vi "LIA Example RT.vi"() -> ()   [LabVIEW 2017]
uses:
  lib/rt/example/Lock-In Amplifier Example RT.lvclass
  <vilib>/userdefined/High Color/nirio_resource_hc.ctl
  lib/rt/example/Properties/Server_GET.vi
  lib/rt/example/Properties/FpgaSession_GET.vi
  lib/rt/server/RT FlexRIO Server TCP.lvclass
  lib/interface/Interface FPGA/LIA Host Interface FPGA.lvclass
panel:
  out "Initialized":bool
  in  "stop":bool
  out "error out":errorcluster
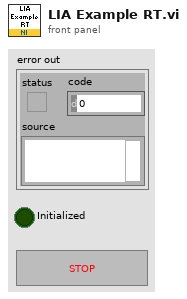
[diagram p1: front panel]
types:
  T1 = typedef "nirio_resource_hc.ctl" = tag
  T2 = typedef "Lock-In Amplifier Example Shared.lvlib/message.ctl" = cluster{"command":u32, "payload":string}
  T3 = typedef "RT FlexRIO Server TCP.lvclass/connection state.ctl" = enum16{"started", "connected", "stopped"}
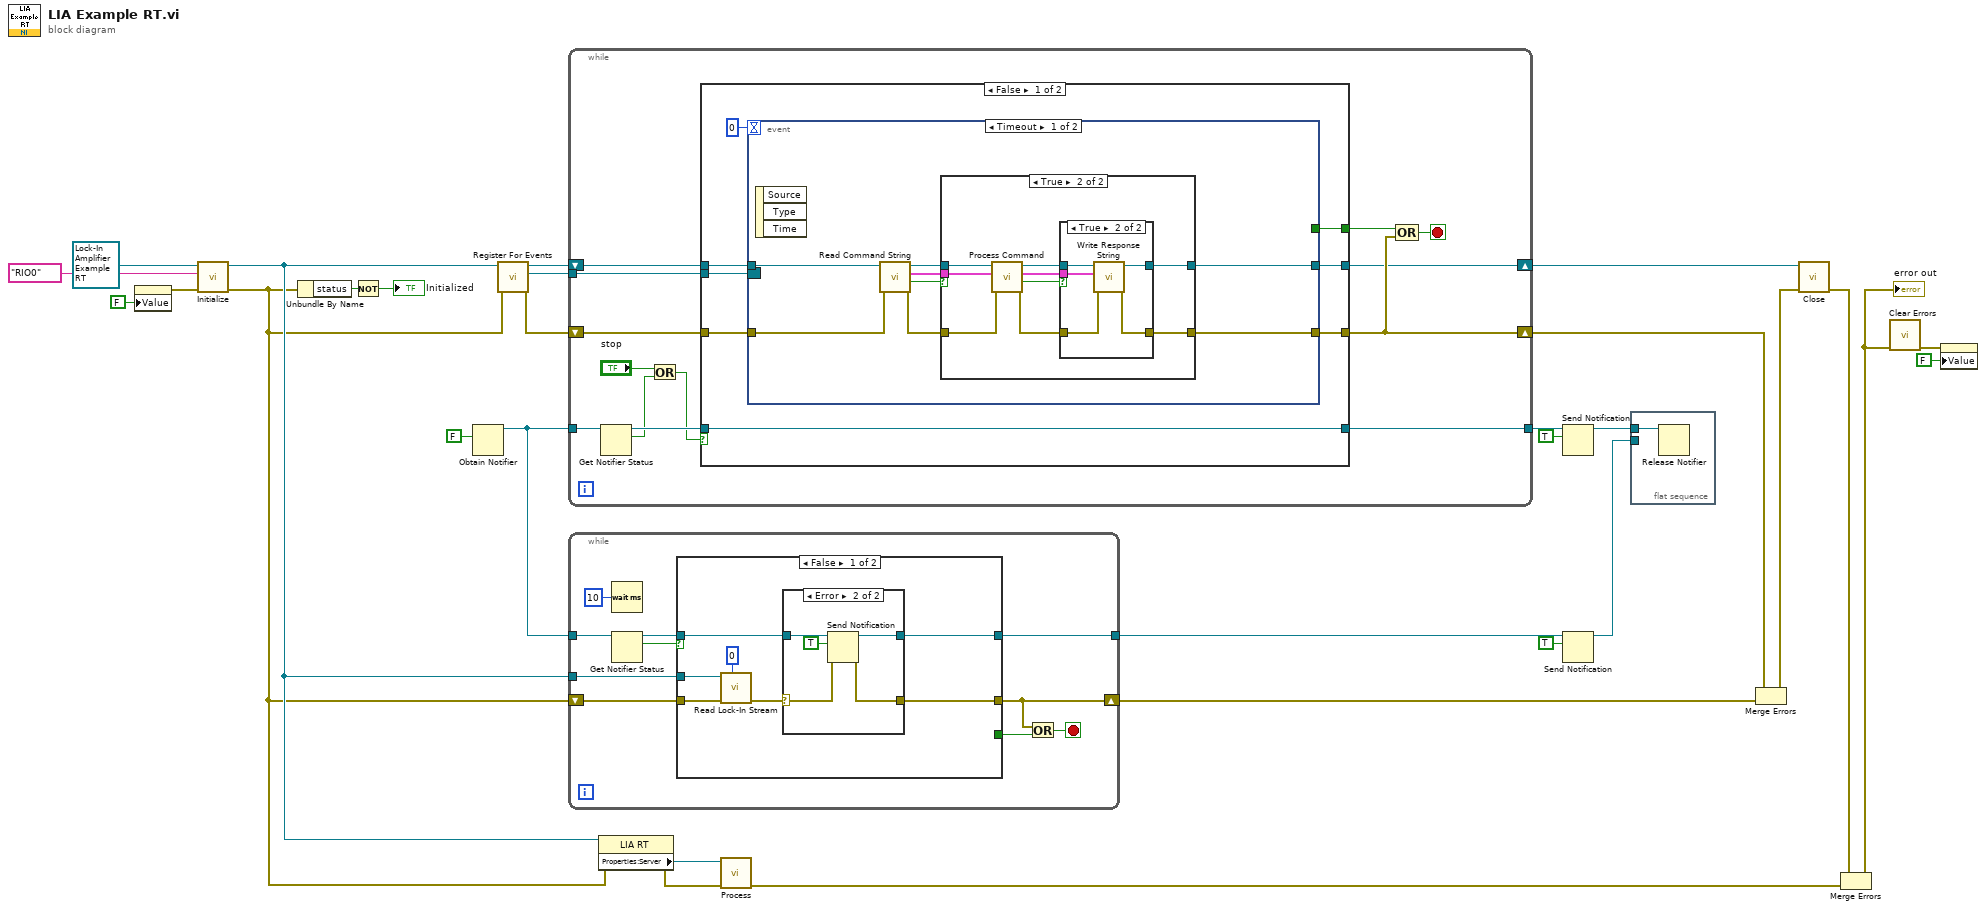
[diagram p0: block diagram]
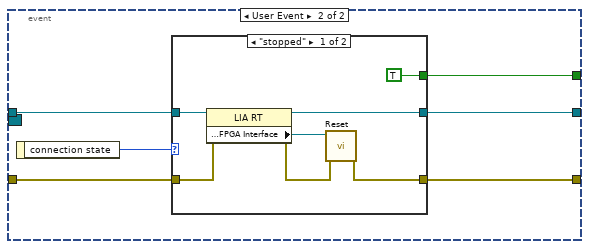
[diagram p4: hidden frame]
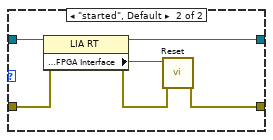
[diagram p5: hidden frame]
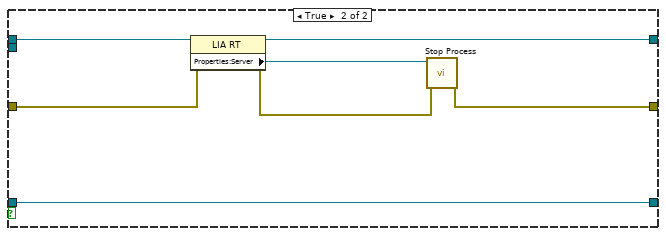
[diagram p6: hidden frame]
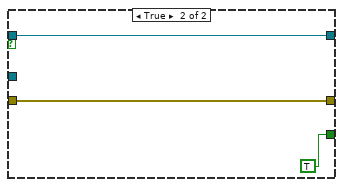
[diagram p8: hidden frame]
diagram:
  n1 = property on="Initialized" class="Bool (strict)"("Value"=FALSE ("Initialized")) -> (error out=w10:errorcluster)  [unwired: 2 in, 1 out]
  n2 = call "Initialize.vi"("error in"=w10, "resource name"=T1 "RIO0", "lia rt in"=refnum<class "Lock-In Amplifier Example RT.lvclass"> refnum) -> ("error out"=w7:errorcluster, "lia rt out"=w8:refnum<class "Lock-In Amplifier Example RT.lvclass">)  [unwired: 7 in]
  n3 = Unbundle By Name(w7) -> ("status"=w6:bool)
  n4 = Not(x=w6) -> (.not. x?=→"Initialized":bool)
  n5 = Obtain Notifier(notification data type=FALSE) -> (notifier out=w28:refnum<notifier>)  [unwired: 3 in, 2 out]
  n6 = call "Register For Events.vi"("error in"=w7, "lia rt in"=w8) -> ("error out"=w15:errorcluster, "event"=w13:refnum<event-registration>, "lia rt out"=w14:refnum<class "Lock-In Amplifier Example RT.lvclass">)  [unwired: 7 in]
  n7 = while {
    shift-right: [w40] -> w3
    shift-left: w15 -> [w41]
    tunnel: w28 -> [w39]
    tunnel: [w38] -> w27
    tunnel: w13 -> [w34]
    shift-right: [w35] -> w19
    shift-left: w14 -> [w42]
    stop <- w43 stop-if-true
    n8 = Get Notifier Status(notifier=w39) -> (notifier out=w37:refnum<notifier>, current notification=w32:bool)  [unwired: 1 in, 3 out]
    n9 = Or(x="stop", y=w32) -> (x .or. y?=w31:bool)
    n10 = case shown="False" w31 {
      tunnel: w42 -> [w51 w101]
      tunnel: w41 -> [w50 w100]
      tunnel: [w49 w98] -> w40
      tunnel: [w48 w103] -> w38
      tunnel: w37 -> [w48 w103]
      tunnel: [w44 _] -> w36
      tunnel: [w47 w99] -> w35
      tunnel: w34 -> [w45 _]
      frame False {
        n11 = event shown="[0] Timeout" {
          selector: w45 -> [_ _]
          dyn-events: _ -> [_ _]
          timeout: 0 -> [_ _]
          tunnel: w51 -> [w59 w83]
          tunnel: w50 -> [w58 w82]
          tunnel: [w57 w80] -> w49
          tunnel: [w56 w81] -> w47
          tunnel: [_ w78] -> w44
          event Timeout {
            n12 = event-data() -> ()  [unwired: 1 in, 3 out]
            n13 = call "Read Command String.vi"("error in"=w58, "lia rt in"=w59) -> ("error out"=w55:errorcluster, "valid"=w52:bool, "message"=w53:T2, "lia rt out"=w54:refnum<class "Lock-In Amplifier Example RT.lvclass">)  [unwired: 6 in]
            n14 = case shown="True" w52 {
              tunnel: w54 -> [w60 w70]
              tunnel: w55 -> [w61 w69]
              tunnel: [w61 w64] -> w57
              tunnel: w53 -> [_ w62]
              tunnel: [w60 w68] -> w56
              frame False {
              }
              frame True {
                n15 = call "Process Command.vi"("error in"=w69, "message in"=w62, "lia rt in"=w70) -> ("error out"=w65:errorcluster, "send response"=w66:bool, "message out"=w63:T2, "lia rt out"=w67:refnum<class "Lock-In Amplifier Example RT.lvclass">)  [unwired: 5 in]
                n16 = case shown="True" w66 {
                  tunnel: [w72 w76] -> w68
                  tunnel: w67 -> [w72 w77]
                  tunnel: w65 -> [w71 w75]
                  tunnel: [w71 w74] -> w64
                  tunnel: w63 -> [_ w73]
                  frame False {
                  }
                  frame True {
                    n17 = call "Write Response String.vi"("error in"=w75, "message in"=w73, "lia rt in"=w77) -> ("error out"=w74:errorcluster, "lia rt out"=w76:refnum<class "Lock-In Amplifier Example RT.lvclass">)  [unwired: 7 in]
                  }
                }
              }
            }
          }
          event User Event {
            n18 = event-data() -> ("connection state"=w79:T3)  [unwired: 1 in]
            n19 = case shown="\"stopped\"" w79 {
              tunnel: w83 -> [w89 w96]
              tunnel: w82 -> [w88 w95]
              tunnel: [w87 w94] -> w81
              tunnel: [w84 w91] -> w80
              tunnel: [TRUE _] -> w78
              frame "stopped" {
                n20 = property class="LIA RT"(reference=w89, error in=w88) -> (reference out=w87:refnum<class "Lock-In Amplifier Example RT.lvclass">, error out=w85:errorcluster, "Properties:FPGA Interface"=w86:refnum<class "LIA Host Interface FPGA.lvclass">)
                n21 = call-dynamic "Reset.vi"("error in"=w85, "host in"=w86) -> ("error out"=w84:errorcluster)  [unwired: 8 in, 1 out]
              }
              frame "started", Default {
                n22 = property class="LIA RT"(reference=w96, error in=w95) -> (reference out=w94:refnum<class "Lock-In Amplifier Example RT.lvclass">, error out=w92:errorcluster, "Properties:FPGA Interface"=w93:refnum<class "LIA Host Interface FPGA.lvclass">)
                n23 = call-dynamic "Reset.vi"("error in"=w92, "host in"=w93) -> ("error out"=w91:errorcluster)  [unwired: 8 in, 1 out]
              }
            }
          }
        }
      }
      frame True {
        n24 = property class="LIA RT"(reference=w101, error in=w100) -> (reference out=w99:refnum<class "Lock-In Amplifier Example RT.lvclass">, error out=w102:errorcluster, "Properties:Server"=w97:refnum<class "RT FlexRIO Server TCP.lvclass">)
        n25 = call "Stop Process.vi"("error in"=w102, "tcp server in"=w97) -> ("error out"=w98:errorcluster)  [unwired: 8 in, 1 out]
      }
    }
    n26 = Compound Arithmetic op=OR(w36, w40) -> (w43:bool)
  }
  n27 = while {
    tunnel: w8 -> [w113]
    tunnel: w28 -> [w111]
    shift-right: [w107] -> w21
    shift-left: w7 -> [w112]
    tunnel: [w109] -> w26
    stop <- w106 stop-if-true
    n28 = Wait (ms)(milliseconds to wait=u32 10) -> ()  [unwired: 1 out]
    n29 = Get Notifier Status(notifier=w111) -> (notifier out=w110:refnum<notifier>, current notification=w108:bool)  [unwired: 1 in, 3 out]
    n30 = case shown="False" w108 {
      tunnel: w113 -> [w120 _]
      tunnel: w112 -> [w119 w129]
      tunnel: w110 -> [w118 w130]
      tunnel: [w116 w129] -> w107
      tunnel: [w115 w130] -> w109
      tunnel: [_ TRUE] -> w105
      frame False {
        n31 = call "Read Lock-In Stream.vi"("instance"=0, "error in"=w119, "lia rt in"=w120) -> ("error out"=w117:errorcluster)  [unwired: 7 in, 1 out]
        n32 = case shown="Error" w117 {
          selector: w117 -> [w121 w126]
          tunnel: w118 -> [w122 w127]
          tunnel: [w121 w125] -> w116
          tunnel: [w122 w123] -> w115
          frame No Error {
          }
          frame Error {
            n33 = Send Notification(notification=TRUE, notifier=w127, error in (no error)=w126) -> (notifier out=w123:refnum<notifier>, error out=w125:errorcluster)
          }
        }
      }
      frame True {
      }
    }
    n34 = Or(x=w107, y=w105) -> (x .or. y?=w106:bool)
  }
  n35 = property class="LIA RT"(reference=w8, error in=w7) -> (error out=w16:errorcluster, "Properties:Server"=w17:refnum<class "RT FlexRIO Server TCP.lvclass">)  [unwired: 1 out]
  n36 = call "Process.vi"("error in"=w16, "server in"=w17) -> ("error out"=w12:errorcluster)  [unwired: 8 in, 1 out]
  n37 = Send Notification(notification=TRUE, notifier=w27) -> (notifier out=w23:refnum<notifier>)  [unwired: 1 in, 1 out]
  n38 = Send Notification(notification=TRUE, notifier=w26) -> (notifier out=w22:refnum<notifier>)  [unwired: 1 in, 1 out]
  n39 = flat-sequence {
    tunnel: w23 -> [w132]
    tunnel: [w131] -> _
    tunnel: w22 -> [w131]
    frame #0 {
      n40 = Release Notifier(notifier=w132) -> ()  [unwired: 2 in, 3 out]
    }
  }
  n41 = Merge Errors(w3, w21) -> (w18:errorcluster)
  n42 = call "Close.vi"("error in"=w18, "lia rt in"=w19) -> ("error out"=w11:errorcluster)  [unwired: 8 in, 1 out]
  n43 = Merge Errors(w11, w12) -> (w2:errorcluster)
  "error out" <- w2
  n44 = call <vilib>:"Clear Errors.vi"("error in (no error)"=w2) -> ("error out"=w1:errorcluster)  [unwired: 5 in, 1 out]
  n45 = property on="Initialized" class="Bool (strict)"(error in=w1, "Value"=FALSE ("Initialized")) -> ()  [unwired: 1 in, 2 out]
